vi "check editor prop nodes.vi"() -> ()   [LabVIEW 2013, in "CVT Consuming Engine Tests.lvlib"]
uses:
  CVT Consuming Engine Tests.lvlib
  <vilib>/NI/Configuration Framework/Node/Summary.ctl
  <vilib>/NI/Configuration Framework/Node/NodeRef.ctl
  <vilib>/NI/Configuration Framework/Node/NISE_CEF_Node.lvclass
  Editor/CVT Engine Editor.lvclass
  <vilib>/NI/Tag Bus Data Framework/Configuration Editor/Classes/Engine Parent/Engine Parent Editor Node.lvclass
  <vilib>/NI/Configuration Framework/serializable configuration/NISE_CEF_serializable configuration.lvclass/NISE_CEF_serializable configuration.ctl
  <vilib>/NI/Configuration Framework/serializable configuration/NISE_CEF_serializable configuration.lvclass
  <vilib>/NI/Configuration Framework/Node/NISE_CEF_Node.lvclass/NISE_CEF_Node.ctl
  <vilib>/NI/Tag Bus Data Framework/Configuration Editor/Classes/Engine Parent/Read Name.vi
  <vilib>/NI/Configuration Framework/serializable configuration/Read UID.vi
  <vilib>/NI/Configuration Framework/Node/ReadChildren.vi
  <vilib>/NI/Configuration Framework/Node/ReadParent.vi
  <vilib>/NI/Tag Bus Data Framework/Configuration Editor/Classes/Engine Parent/read engine configuration.vi
  <vilib>/NI/Configuration Framework/serializable configuration/get alias.vi
  <vilib>/NI/Configuration Framework/Node/ReadNodeClass.vi
  <vilib>/NI/Module Execution Interface/Engine Configuration/engine configuration.lvclass
panel:
  out "Name":string
  out "UID 2":string
  out "error out 3":errorcluster
  out "visible":bool
  out "is abstract":bool
  out "error out 2":errorcluster
  out "UID":string
  out "Parent":T1
  out "NodeClass":string
  out "Children":T1[](array[typedef])
  out "error out":errorcluster
  out "summary":T2[](array[typedef])
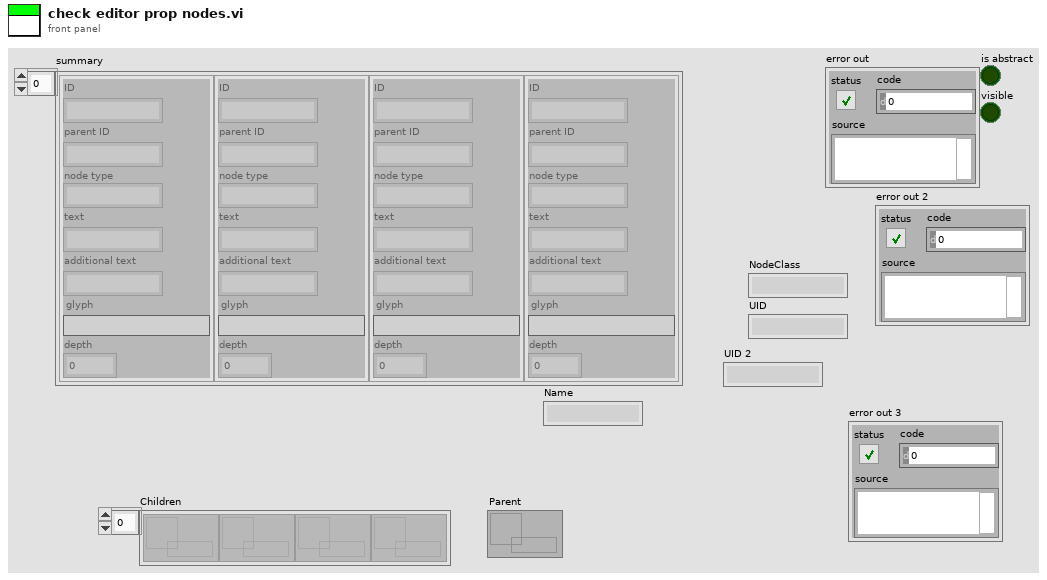
[diagram p1: front panel]
types:
  T1 = typedef "NISE_CEF_Node.lvclass/NodeRef.ctl" = refnum<data-value>
  T2 = typedef "NISE_CEF_Node.lvclass/Summary.ctl" = cluster{"ID":string, "parent ID":string, "node type":string, "text":string, "additional text":string, "glyph":string, "depth":i32}
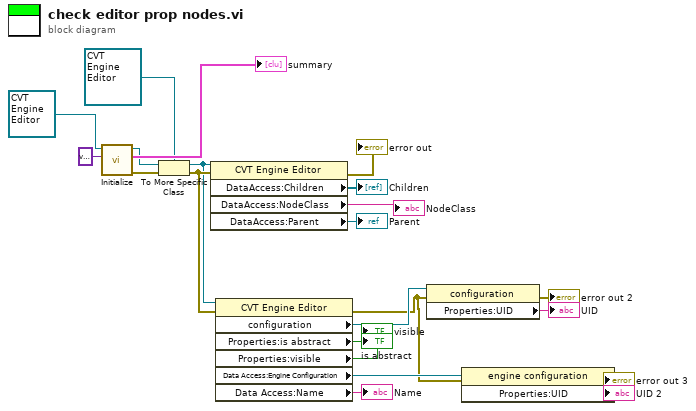
[diagram p0: block diagram]
diagram:
  n1 = call-dynamic "Initialize.vi"("parameters"=variant, "Engine in"=refnum<class "CVT Engine Editor.lvclass"> refnum ("CVT Engine Editor")) -> ("error out"=w19:errorcluster, "summary"=→"summary":T2[], "data value reference"=w18:T1)  [unwired: 7 in]
  n2 = To More Specific Class(target class=refnum<data-value> refnum, reference=w18, error in=w19) -> (specific class reference=w11:refnum<data-value>, error out=w12:errorcluster)
  n3 = property class="CVT Engine Editor"(reference=w11, error in=w12) -> (error out=→"error out":errorcluster, "DataAccess:Children"=→"Children":T1[], "DataAccess:NodeClass"=→"NodeClass":string, "DataAccess:Parent"=→"Parent":T1)  [unwired: 1 out]
  n4 = property class="CVT Engine Editor"(reference=w11, error in=w12) -> (error out=w2:errorcluster, "configuration"=w10:refnum<class "NISE_CEF_serializable configuration.lvclass">, "Properties:is abstract"=→"is abstract":bool, "Properties:visible"=→"visible":bool, "Data Access:Engine Configuration"=w3:refnum<class "engine configuration.lvclass">, "Data Access:Name"=→"Name":string)  [unwired: 1 out]
  n5 = property class="configuration"(reference=w10, error in=w2) -> (error out=→"error out 2":errorcluster, "Properties:UID"=→"UID":string)  [unwired: 1 out]
  n6 = property class="engine configuration"(reference=w3, error in=w2) -> (error out=→"error out 3":errorcluster, "Properties:UID"=→"UID 2":string)  [unwired: 1 out]
